vi "AKIP_set_parameters.vi"(8 "error in (no error)":errorcluster, 11 "VISA Refnum in":refnum<visa-resource-name>) -> (0 "error out":errorcluster, 3 "VISA Refnum out":refnum<visa-resource-name>)   [LabVIEW 2017]
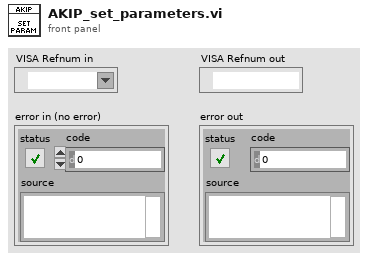
[diagram p1: front panel]
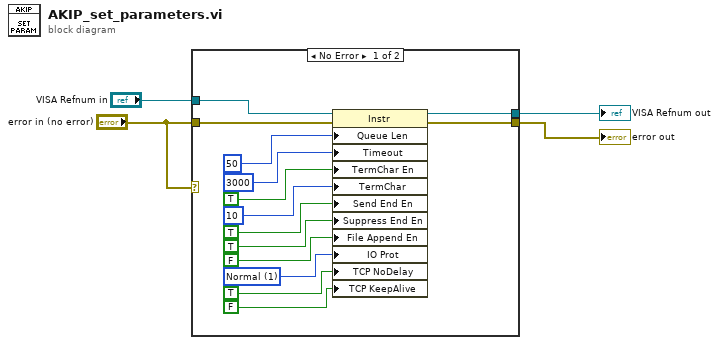
[diagram p0: block diagram]
diagram:
  n1 = case shown="No Error" "error in (no error)" {
    tunnel: "error in (no error)" -> [w8 w19]
    tunnel: "VISA Refnum in" -> [w7 w20]
    tunnel: [w6 w19] -> w3
    tunnel: [w5 w20] -> w2
    frame No Error {
      w16 = u16 1 items=["Normal"=1, "VXI/FDC"=2, "GPIB/HS488"=3, "Serial-TCPIP-USB/488 Strings"=4, "USBTMC/Vendor-Specific"=5] ("Message Based Settings:IO Protocol")
      n2 = property class="Instr"(reference=w7, error in=w8, "Queue Len"=u32 50 ("General Settings:Maximum Queue Length"), "Timeout"=u32 3000 ("General Settings:Timeout Value"), "TermChar En"=TRUE ("Message Based Settings:Termination Character Enable"), "TermChar"=u8 10 ("Message Based Settings:Termination Character"), "Send End En"=TRUE ("Message Based Settings:Send End Enable"), "Suppress End En"=TRUE ("Message Based Settings:Suppress End Enable"), "File Append En"=FALSE ("Message Based Settings:File Append Enable"), "IO Prot"=w16, "TCP NoDelay"=TRUE ("TCP/IP Settings:No Packet Delay"), "TCP KeepAlive"=FALSE ("TCP/IP Settings:Keep-Alive Packets")) -> (reference out=w5:refnum<visa-resource-name>, error out=w6:errorcluster)
    }
    frame Error {
    }
  }
  "error out" <- w3
  "VISA Refnum out" <- w2
